vi "Build Type to Names.vi"(8 "error in (no error)":errorcluster, 10 "Build Type String":string, 11 "Library Name":string) -> (0 "error out":errorcluster, 1 "Package Name":string, 2 "PROVIDES/DEPENDS Name":string, 3 "Display Name":string)   [LabVIEW 2019, in "NIPKG Naming.lvlib"]
uses:
  NIPKG Naming.lvlib
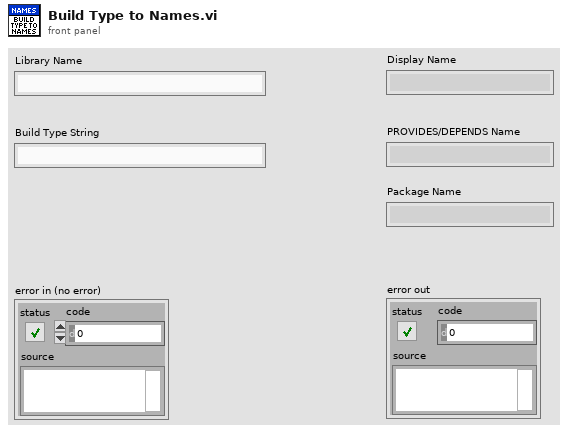
[diagram p1: front panel]
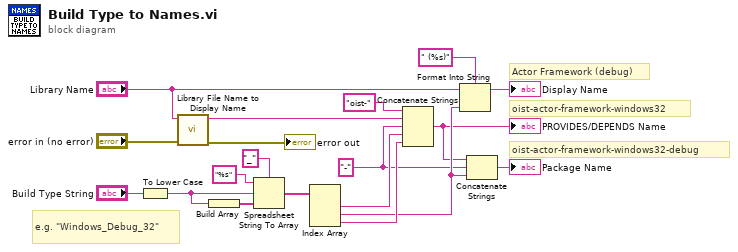
[diagram p0: block diagram]
diagram:
  w11 = "-" ("replace string (\"\")")
  # "Actor Framework (debug)"
  # "oist-actor-framework-windows32-debug"
  # "oist-actor-framework-windows32"
  # "e.g. \"Windows_Debug_32\""
  n1 = To Lower Case(string="Build Type String") -> (all lower case string=w12:string)
  n2 = call "Library File Name to Display Name.vi"("error in (no error)"="error in (no error)", "Library Name"="Library Name") -> ("error out"=→"error out":errorcluster, "Display Name"=w7:string)  [unwired: 8 in]
  n3 = Build Array(w12) -> (w15:string[])
  n4 = Spreadsheet String To Array(delimiter (Tab)="_", format string="%s", spreadsheet string=w12, array type (2D Dbl)=w15) -> (array=w14:string[])
  n5 = Index Array(array=w14) -> (element #1=w13:string, element #2=w18:string, element #3=w19:string)  [unwired: 3 in]
  n6 = Concatenate Strings("oist-" ("string"), w7, w11, w13, w19) -> (w10:string)
  "PROVIDES/DEPENDS Name" <- w10
  n7 = Format Into String(format string=" (%s)", initial string="Library Name", w18) -> (resulting string=→"Display Name":string)  [unwired: 1 in, 1 out]
  n8 = Concatenate Strings(w10, w11, w18) -> (→"Package Name":string)
